vi "movingInTurnState.vi"(0 "KickToSkill in":refnum<class "KickToSkill.lvclass">, 5 "Target":dbl[](array[numeric]), 7 "Robot":refnum<class "Robot.lvclass">, 9 "RobotRef":refnum<class "Robot.lvclass">[](array[class]), 11 "error in (no error)":errorcluster, 12 "first call":bool, 13 "DistFromEnemyToConsider\nMoveInTurnState":dbl) -> (4 "KickToSkill out":refnum<class "KickToSkill.lvclass">, 6 "Dest":dbl[](array[numeric]), 8 "RobotToClose":bool, 15 "error out":errorcluster)   [LabVIEW 2020, in "KickToSkill.lvclass"]
uses:
  KickToSkill.lvclass
  Robot_class/Robot.lvclass
  C:/Users/anton/Desktop/RoboIME/SSL_COMP/SSL_AI/Object_class/Object.lvclass
  Object_class/Object.lvclass/Object.ctl
  Robot_class/Robot.lvclass/Robot.ctl
  <vilib>/Analysis/coordinate.llb/2D Cartesian Coordinate Rotation (Scalar).vi
  <vilib>/Analysis/baseanly.llb/Unit Vector (DBL).vi
  Robot_class/Read id.vi
  Object_class/Read position(x,y).vi
  Utilities_class/Utilities.lvclass
  <vilib>/Analysis/NI_AALPro.lvlib
  <vilib>/Analysis/NI_AALBase.lvlib
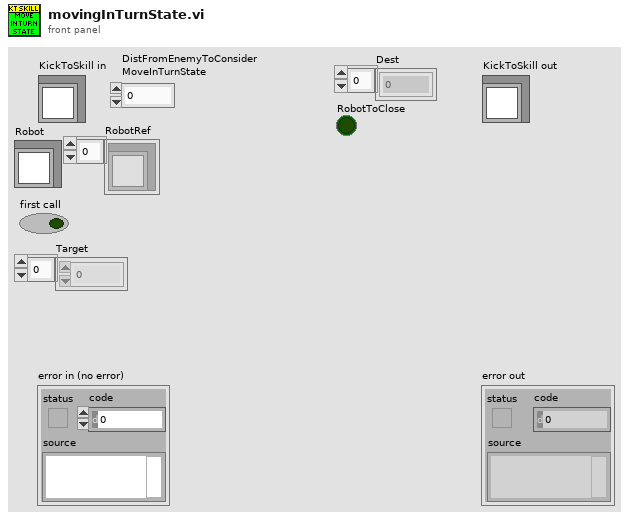
[diagram p1: front panel]
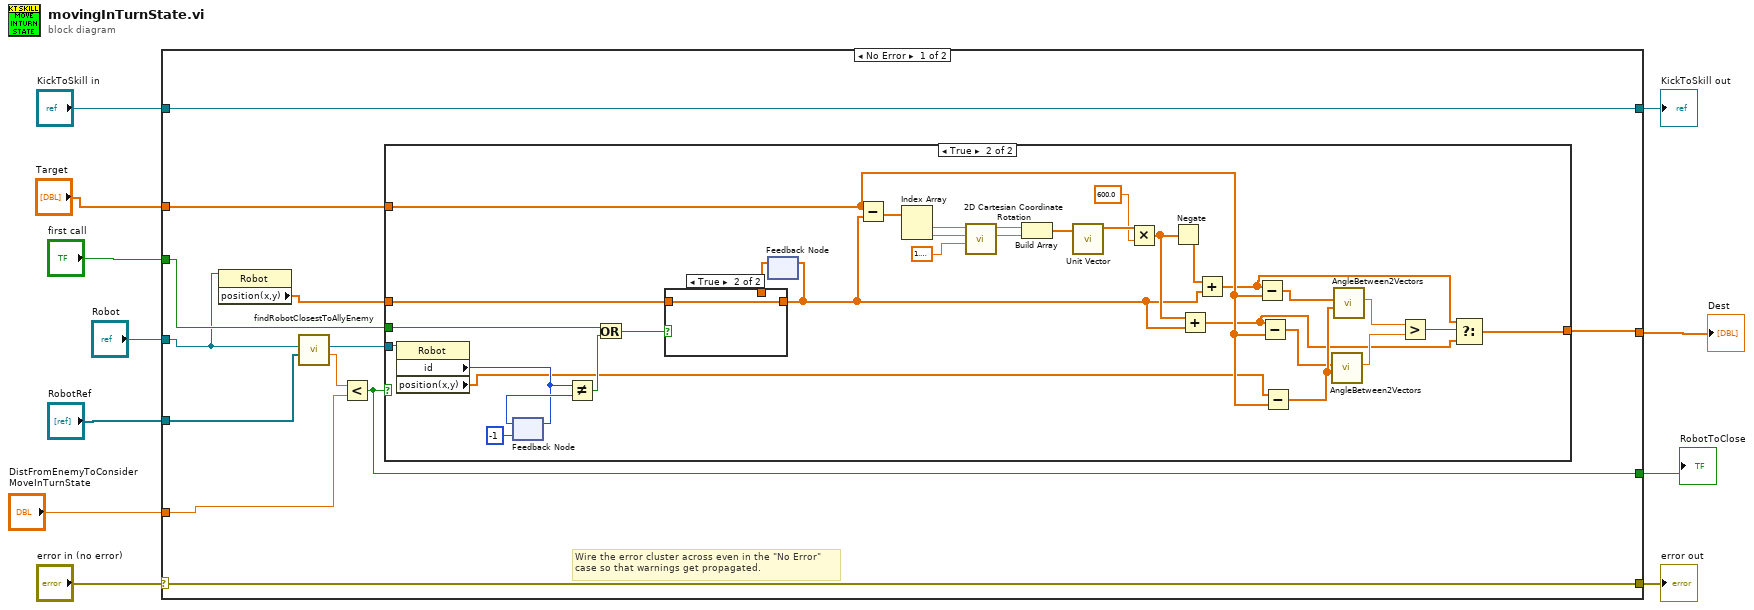
[diagram p0: block diagram]
diagram:
  n1 = case shown="No Error" "error in (no error)" {
    selector: "error in (no error)" -> [w22 w60]
    tunnel: [w22 w60] -> w10
    tunnel: [w23 w59] -> w8
    tunnel: "KickToSkill in" -> [w23 w59]
    tunnel: "Robot" -> [w18 _]
    tunnel: "RobotRef" -> [w21 _]
    tunnel: "first call" -> [w19 _]
    tunnel: "Target" -> [w16 _]
    tunnel: [w15 _] -> w3
    tunnel: [w13 _] -> w2
    tunnel: "DistFromEnemyToConsider\nMoveInTurnState" -> [w12 _]
    frame No Error {
      # "Wire the error cluster across even in the \"No Error\"\ncase so that warnings get propagated."
      n2 = property class="Robot"(reference=w18) -> ("position(x,y)"=w17:dbl[])  [unwired: 1 in, 2 out]
      n3 = call "findRobotClosestToAllyEnemy.vi"("Ally/Enemy Robots"=w21, "Robot Target"=w18) -> ("Robot distance to other one"=w14:dbl, "Robot"=w20:refnum<class "Robot.lvclass">)  [unwired: 6 in, 2 out]
      n4 = Less?(x=w14, y=w12) -> (x < y?=w13:bool)
      n5 = case shown="True" w13 {
        tunnel: w20 -> [_ w56]
        tunnel: w19 -> [_ w55]
        tunnel: w17 -> [w24 w49]
        tunnel: w16 -> [_ w35]
        tunnel: [w24 w25] -> w15
        frame False {
        }
        frame True {
          n6 = property class="Robot"(reference=w56) -> ("id"=w53:i32, "position(x,y)"=w34:dbl[])  [unwired: 1 in, 2 out]
          n7 = feedback #1(-1 ("id")) -> (w54:i32)
          n8 = feedback-in #1(w53) -> ()
          n9 = Not Equal?(x=w53, y=w54) -> (x != y?=w51:bool)
          n10 = Or(x=w55, y=w51) -> (x .or. y?=w50:bool)
          n11 = feedback #2() -> (w48:dbl[])  [unwired: 1 in]
          n12 = case shown="True" w50 {
            tunnel: w49 -> [_ w58]
            tunnel: [w57 w58] -> w36
            tunnel: w48 -> [w57 _]
            frame False {
            }
            frame True {
            }
          }
          n13 = feedback-in #2(w36) -> ()
          n14 = Subtract(x=w35, y=w36) -> (x-y=w47:dbl[])
          n15 = Index Array(array=w47) -> (element #1=w46:dbl, element #2=w45:dbl)  [unwired: 2 in]
          n16 = call-poly <vilib>:"2D Cartesian Coordinate Rotation.vi"("theta"=1.5707963267948966, "y"=w45, "x"=w46) -> ("y out"=w42:dbl, "x out"=w43:dbl)  [unwired: 6 in, 1 out]
          n17 = Build Array(w43, w42) -> (w41:dbl[])
          n18 = call-poly <vilib>:"Unit Vector.vi"("Input Vector"=w41) -> ("Unit Vector"=w40:dbl[])  [unwired: 8 in, 2 out]
          n19 = Multiply(x=w40, y=600.0) -> (x*y=w37:dbl[])
          n20 = Negate(x=w37) -> (-x=w38:dbl[])
          n21 = Add(x=w37, y=w36) -> (x+y=w26:dbl[])
          n22 = Add(x=w38, y=w36) -> (x+y=w27:dbl[])
          n23 = Subtract(x=w27, y=w35) -> (x-y=w32:dbl[])
          n24 = Subtract(x=w26, y=w35) -> (x-y=w31:dbl[])
          n25 = Subtract(x=w34, y=w35) -> (x-y=w33:dbl[])
          n26 = call "AngleBetween2Vectors.vi"("Array 1"=w33, "Array 2"=w31) -> ("angleInRadians(default)"=w29:dbl)  [unwired: 6 in, 3 out]
          n27 = call "AngleBetween2Vectors.vi"("Array 1"=w33, "Array 2"=w32) -> ("angleInRadians(default)"=w30:dbl)  [unwired: 6 in, 3 out]
          n28 = Greater?(x=w30, y=w29) -> (0:w28:bool)
          n29 = Select(t=w27, s=w28, f=w26) -> (s? t:f=w25:dbl[])
        }
      }
    }
    frame Error {
    }
  }
  "error out" <- w10
  "KickToSkill out" <- w8
  "Dest" <- w3
  "RobotToClose" <- w2
